vi "ACP Configure Common.vi"(7 "Selector String":string, 8 "error in (no error)":errorcluster, 10 "ACP Common Configuration":T1={"Averaging Count"=10, "Averaging Enabled"=0, "Averaging Type"=0, "FFT Padding"=1.0, "FFT Window"=1, "Sweep Time Interval (s)"=0.001, "Sweep Time Auto"=1, "RBW Filter Type"=1, "RBW (Hz)"=10000.0, "RBW Auto"=1, "Power Units"=0} {"Power Units" items=["dBm", "dBm/Hz"]; "RBW Auto" items=["False", "True"]; "RBW (Hz)" format="%.3p"; "RBW Filter Type" items=["FFT Based", "Gaussian", "Flat", "Synch Tuned - 4", "Synch Tuned - 5"]; "Sweep Time Auto" items=["False", "True"]; "Sweep Time Interval (s)" format="%.2p"; "FFT Window" items=["None", "Flat Top", "Hanning", "Hamming", "Gaussian", "Blackman", "Blackman-Harris", "Kaiser-Bessel"]; "FFT Padding" format="%.2f"; "Averaging Type" items=["RMS", "Log", "Scalar", "Max", "Min", "Vector"]; "Averaging Enabled" items=["False", "True"]}, 11 "Instrument Handle In":refnum<k21>) -> (0 "error out":errorcluster, 3 "Instrument Handle Out":refnum<k21>)   [LabVIEW 2016, in "RFmxSpecAn.lvlib"]
uses:
  RFmxSpecAn.lvlib
  Typedefs/ACP Common Configuration.ctl
  <resource>/objmgr/RFmxSpecAn.rc
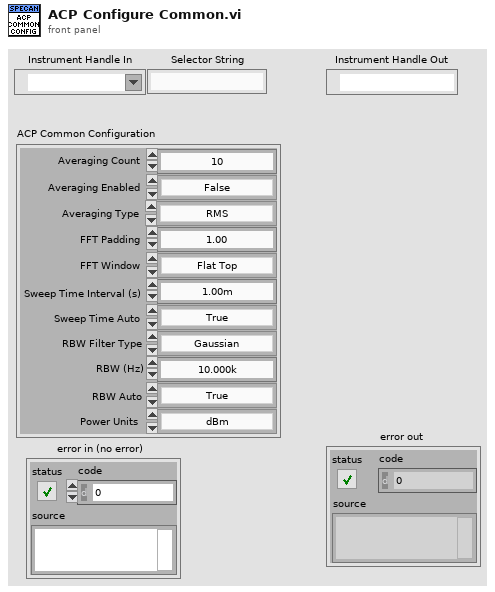
[diagram p1: front panel]
types:
  T1 = typedef "RFmxSpecAn.lvlib/ACP Common Configuration.ctl" = cluster{"Averaging Count":i32, "Averaging Enabled":i32, "Averaging Type":i32, "FFT Padding":dbl, "FFT Window":i32, "Sweep Time Interval (s)":dbl, "Sweep Time Auto":i32, "RBW Filter Type":i32, "RBW (Hz)":dbl, "RBW Auto":i32, "Power Units":i32}
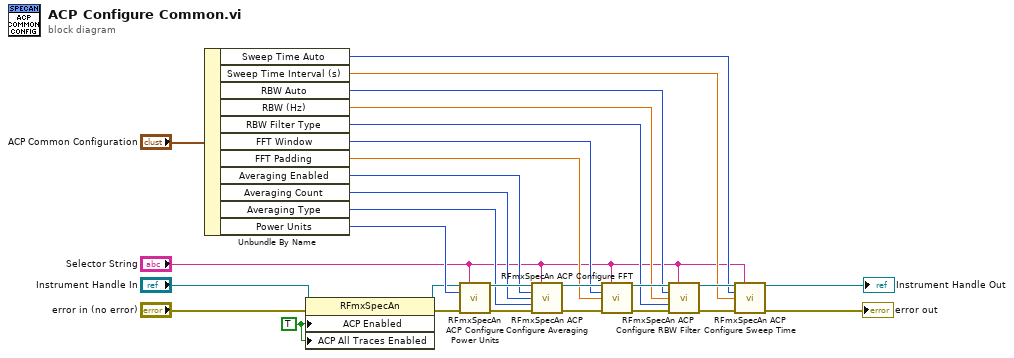
[diagram p0: block diagram]
diagram:
  w4 = TRUE ("ACP Enabled")
  n1 = Unbundle By Name("ACP Common Configuration") -> ("Sweep Time Auto"=w10:i32, "Sweep Time Interval (s)"=w9:dbl, "RBW Auto"=w11:i32, "RBW (Hz)"=w12:dbl, "RBW Filter Type"=w13:i32, "FFT Window"=w15:i32, "FFT Padding"=w14:dbl, "Averaging Enabled"=w18:i32, "Averaging Count"=w17:i32, "Averaging Type"=w16:i32, "Power Units"=w19:i32)
  n2 = property class="RFmxSpecAn"(reference="Instrument Handle In", error in="error in (no error)", "ACP Enabled"=w4, "ACP All Traces Enabled"=w4) -> (reference out=w5:refnum<k21>, error out=w7:errorcluster)
  n3 = call <vilib>:"RFmxSpecAn ACP Configure Power Units.vi"("Instrument Handle In"=w5, "Selector String"="Selector String", "Power Units"=w19, "error in (no error)"=w7) -> ("Instrument Handle Out"=w24:refnum<k21>, "error out"=w23:errorcluster)  [unwired: 10 in]
  n4 = call <vilib>:"RFmxSpecAn ACP Configure Averaging.vi"("Instrument Handle In"=w24, "Selector String"="Selector String", "Averaging Enabled"=w18, "Averaging Count"=w17, "Averaging Type"=w16, "error in (no error)"=w23) -> ("Instrument Handle Out"=w22:refnum<k21>, "error out"=w28:errorcluster)  [unwired: 8 in]
  n5 = call <vilib>:"RFmxSpecAn ACP Configure FFT.vi"("Instrument Handle In"=w22, "Selector String"="Selector String", "FFT Window"=w15, "FFT Padding"=w14, "error in (no error)"=w28) -> ("Instrument Handle Out"=w26:refnum<k21>, "error out"=w25:errorcluster)  [unwired: 9 in]
  n6 = call <vilib>:"RFmxSpecAn ACP Configure RBW Filter.vi"("Instrument Handle In"=w26, "Selector String"="Selector String", "RBW Auto"=w11, "RBW (Hz)"=w12, "RBW Filter Type"=w13, "error in (no error)"=w25) -> ("Instrument Handle Out"=w21:refnum<k21>, "error out"=w27:errorcluster)  [unwired: 8 in]
  n7 = call <vilib>:"RFmxSpecAn ACP Configure Sweep Time.vi"("Instrument Handle In"=w21, "Selector String"="Selector String", "Sweep Time Auto"=w10, "Sweep Time Interval (s)"=w9, "error in (no error)"=w27) -> ("Instrument Handle Out"=→"Instrument Handle Out":refnum<k21>, "error out"=→"error out":errorcluster)  [unwired: 9 in]
